vi "VerticalButtonBar_Create.vi"(8 "ErrorIn":errorcluster, 11 "ReferenceIn":refnum<class "VerticalButtonBar.lvclass">) -> (0 "ErrorOut":errorcluster, 3 "ReferenceOut":refnum<class "VerticalButtonBar.lvclass">)   [LabVIEW 2021, in "VerticalButtonBar.lvclass"]
uses:
  VerticalButtonBar.lvclass
  C:/Localdata/Projects/TriekselSoft/TriekselsoftApplicationFramework/Source/.Externals/Library_TAF_ApplicationFramework/TAFBaseGUI/TAFBaseGUI.lvclass
  VerticalButtonBar.lvclass/VerticalButtonBar.ctl
  Library_TAF_ApplicationFramework/TAFBaseGUI/TAFBaseGUI.lvclass
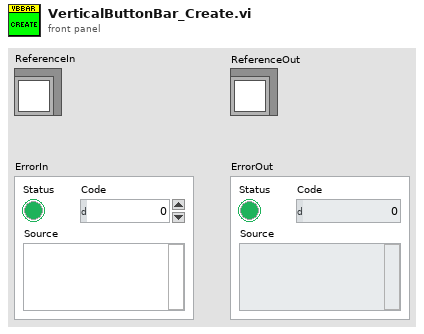
[diagram p1: front panel]
types:
  T1 = typedef "VerticalButtonBar.lvclass/ObjectAttributes.ctl" = cluster{"Interfaces":cluster{"IDockGUI":refnum<class "IDockGUI.lvclass">, "Authorizer":refnum<class "IAuthorization.lvclass">}, "Locals":cluster{"ButtonBar":refnum<class "ButtonCollection.lvclass">, "BaseConfigurationPath":path, "Labels":cluster{"Label":string, "Value":string}[]}, "Persistent":cluster{"ButtonDefinitionFile":string}}
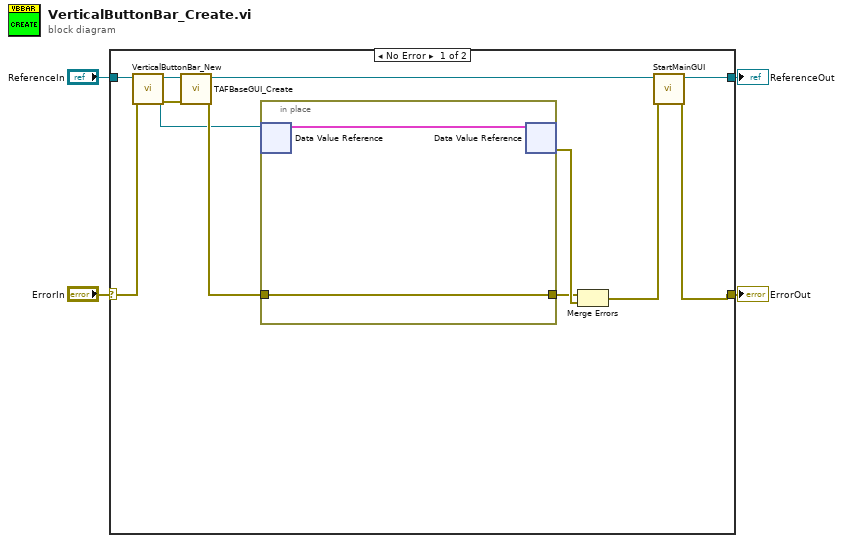
[diagram p0: block diagram]
diagram:
  n1 = case shown="No Error" "ErrorIn" {
    selector: "ErrorIn" -> [w13 w20]
    tunnel: [w10 w20] -> w3
    tunnel: "ReferenceIn" -> [w9 w19]
    tunnel: [w5 w19] -> w1
    frame No Error {
      n2 = call "VerticalButtonBar_New.vi"("ErrorIn"=w13, "ReferenceIn"=w9) -> ("ErrorOut"=w12:errorcluster, "DVRRefOut"=w7:refnum<data-value>, "ReferenceOut"=w8:refnum<class "VerticalButtonBar.lvclass">)  [unwired: 6 in, 1 out]
      n3 = call "TAFBaseGUI_Create.vi"("ErrorIn"=w12, "ReferenceIn"=w8) -> ("ErrorOut"=w15:errorcluster, "ReferenceOut"=w6:refnum<class "VerticalButtonBar.lvclass">)  [unwired: 8 in]
      n4 = in-place {
        in-place-border: w15 -> [w18]
        in-place-border: [w18] -> w14
        n5 = in-place-dvr #1(w7) -> (w17:T1)  [unwired: 1 out]
        n6 = in-place-dvr #1(w17) -> (w16:errorcluster)  [unwired: 1 out]
      }
      n7 = Merge Errors(w14, w16) -> (w11:errorcluster)
      n8 = call "StartMainGUI.vi"("ErrorIn"=w11, "ReferenceIn"=w6) -> ("ErrorOut"=w10:errorcluster, "ReferenceOut"=w5:refnum<class "VerticalButtonBar.lvclass">)  [unwired: 6 in, 2 out]
    }
    frame Error {
      # "VI-TechBaseTemplate_Simple_4x4x4"
    }
  }
  "ErrorOut" <- w3
  "ReferenceOut" <- w1
